vi "KH TURCK ETHERNETIP Global.vi"() -> ()   [LabVIEW 2017]
uses:
  KH TURCK ETHERNETIP TDefCluster TBEN-S2-4AI Input Values.ctl
  KH TURCK ETHERNETIP TDefCluster TBEN-S1-8DXP Input Values.ctl
  KH TURCK ETHERNETIP TDefCluster TBEN-S2-2RFID-4DXP Input Values.ctl
  KH TURCK ETHERNETIP TDefCluster TBEN-S2-4AO Input Values.ctl
  KH TURCK ETHERNETIP TDef Enum IOL Data.ctl
panel:
  in  "Tab Control 2":enum32{"AI", "DXP", "RFID", "AO", "IOL"}(tab)
  out "Read AI":T1[](array[typedef])
  out "Read DXP":T2[](array[typedef])
  out "RFID_Read":T3[](array[typedef])
  out "Data Turck":u8[](array[numeric]) format="%.0x"
  out "Read AO":T4[](array[typedef])
  out "Read IOL":T5[](array[typedef])
  # "Wire Break"
  # "upper limit"
  # "Overflow"
  # "Underflow"
  # "CJC Wire Break"
  # "Overcurrent (RTD)"
  # "Overcurrent supply VAUX1"
  # "Lower limit value underrun"
  # "Ch0"
  # "Ch1"
  # "Ch2"
  # "Ch3"
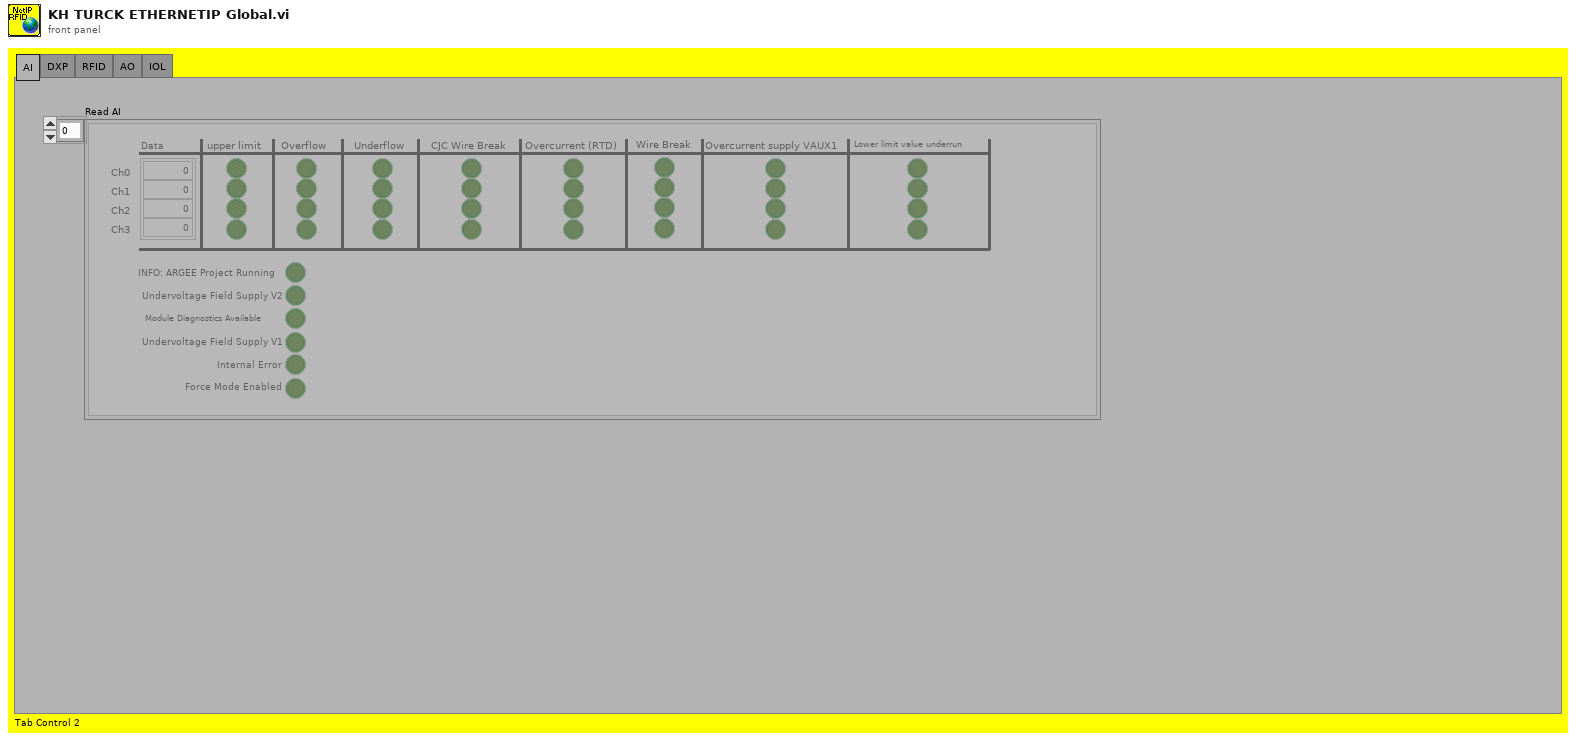
[diagram p1: front panel]
types:
  T1 = typedef "KH TURCK ETHERNETIP TDefCluster TBEN-S2-4AI Input Values.ctl" = cluster{"Data":i16[], "upper Limit CH0":bool, "upper Limit CH1":bool, "upper Limit CH2":bool, "upper Limit CH3":bool, "Overflow CH0":bool, "Overflow CH1":bool, "Overflow CH2":bool, "Overflow CH3":bool, "Underflow CH0":bool, "Underflow CH1":bool, "Underflow CH2":bool, "Underflow CH3":bool, "CJC Wire Break CH0":bool, "CJC Wire Break CH1":bool, "CJC Wire Break CH2":bool, "CJC Wire Break CH3":bool, "Overcurrent (RTD) CH0":bool, "Overcurrent (RTD) CH1":bool, "Overcurrent (RTD) CH2":bool, "Overcurrent (RTD) CH3":bool, "Wire Break CH0":bool, "Wire Break CH1":bool, "Wire Break CH2":bool, "Wire Break CH3":bool, "Overcurrent supply VAUX1 CH0":bool, "Overcurrent supply VAUX1 CH1":bool, "Overcurrent supply VAUX1 CH2":bool, "Overcurrent supply VAUX1 CH3":bool, "Lower limit value underrun CH0":bool, "Lower limit value underrun CH1":bool, "Lower limit value underrun CH2":bool, "Lower limit value underrun CH3":bool, "Module Diagnostics Available":bool, "INFO: ARGEE Project Running":bool, "Undervoltage Field Supply V2":bool, "Undervoltage Field Supply V1":bool, "Internal Error":bool, "Force Mode Enabled":bool}
  T2 = typedef "KH TURCK ETHERNETIP TDefCluster TBEN-S1-8DXP Input Values.ctl" = cluster{"Data":bool[], "Overcurrent":bool[], "Overcurrent VAUX1 Ch0-3":bool, "Overcurrent VAUX2 Ch4-7":bool, "Latch Input":bool[], "Counter value":u32, "Counter frequency (Hz)":u16, "Status":u8, "Overcurrent PWM Output 3":u8, "Overcurrent PWM Output 7":u8, "Module Diagnostics Available":bool, "INFO: ARGEE Project Running":bool, "Undervoltage V2":bool, "Undervoltage V1":bool, "Force Mode Enabled":bool}
  T3 = typedef "KH TURCK ETHERNETIP TDefCluster TBEN-S2-2RFID-4DXP Input Values.ctl" = cluster{"Station Status Word (Input Data Mapping)":cluster{"Module diagnostics avaliable":bool, "INFO: ARGEE Project Running":bool, "Undervoltage V2":bool, "Undervoltage V1":bool, "Internal Error":bool, "I/O-ASSISTANT Force Mode active":bool}, "RFID control/status 0 (Input Data Mapping)":cluster{"Tag present at r/w head":bool[], "response code":u16, "loop counter":u8, "Length":u16, "Error code":u16, "Tag counter":u16, "Data (Bytes) available":u16, "Read fragment No.":u8, "Write fragment No.":u8, "Tag present at r/w head bit":bool, "HF r/w head switched on":bool, "Continuous mode active":bool, "Antenna detuned at HF read/write head":bool, "Parameter not supported by read/write head":bool, "Error reported by read/write head":bool, "Not connected to read/write head":bool}, "RFID read data 0 (Input Data Mapping)":u8[], "RFID control/status 1 (Input Data Mapping)":cluster{"response code":u16, "Loop counter":u8, "Length":u16, "Error code":u16, "Tag counter":u16, "Data (Bytes) available":u16, "Read fragment No.":u8, "Write fragment No.":u8, "Tag present at r/w head bit":bool, "HF r/w head switched on":bool, "Continuous mode active":bool, "Antenna detuned at HF read/write head":bool, "Parameter not supported by read/write head":bool, "Error reported by read/write head":bool, "Not connected to read/write head":bool, "Tag present at r/w head":bool[]}, "RFID read data 1 (Input Data Mapping)":u8[], "RFID diagnostics (Input Data Mapping)":cluster{"Overcurrent supply VAUX1 (a)":bool, "Parameterization error (a)":bool, "Configuration via DTM active (a)":bool, "Buffer full (a)":bool, "Antenna detuned at HF read/write head (a)":bool[], "Parameter not supported by read/write head (a)":bool[], "Error reported by read/write head (a)":bool[], "Not connected to read/write head (a)":bool[], "Overcurrent supply VAUX1 (b)":bool, "Parameterization error (b)":bool, "Configuration via DTM active (b)":bool, "Buffer full (b)":bool, "Antenna detuned at HF read/write head (b)":bool[], "Parameter not supported by read/write head (b)":bool[], "Error reported by read/write head (b)":bool[], "Not connected to read/write head (b)":bool[]}, "DXP diagnostics (Input Data Mapping)":cluster{"Overcurrent VAUX2 Ch4/5":bool, "Overcurrent VAUX2 Ch6/7":bool, "Channel 4 - Output overcurrent":bool, "Channel 5 - Output overcurrent":bool, "Channel 6 - Output overcurrent":bool, "Channel 7 - Output overcurrent":bool}, "DXP (Input Data Mapping)":cluster{"Channel 4 - Input value":bool, "Channel 5 - Input value":bool, "Channel 6 - Input value":bool, "Channel 7 - Input value":bool}}
  T4 = typedef "KH TURCK ETHERNETIP TDefCluster TBEN-S2-4AO Input Values.ctl" = cluster{"Overload Ch0":bool, "Overload Ch1":bool, "Overload Ch2":bool, "Overload Ch3":bool, "Wirebreak Ch0":bool, "Wirebreak Ch1":bool, "Wirebreak Ch2":bool, "Wirebreak Ch3":bool, "Module Diagnostics Available":bool, "INFO: ARGEE Project Running":bool, "Undervoltage V2":bool, "Undervoltage V1":bool, "Internal Error":bool, "Force Mode Enabled":bool}
  T5 = typedef "KH TURCK ETHERNETIP TDef Enum IOL Data.ctl" = cluster{"Data_Port1":u16[], "Data_Port2":u16[], "Data_Port3":u16[], "Data_Port4":u16[], "Status":cluster{"Undervoltage Field Supply V2":bool, "Overvoltage Field Supply V1":bool, "Undervoltage Field Supply V1":bool, "Internal Error":bool, "Module Diagnostics Available":bool, "Station Configuration Changed":bool, "Overcurrent Isys":bool, "Overvoltage Field Supply V2":bool, "Force Mode Enabled":bool}, "Diagnostics":cluster{"Channel 2 - Output signal overcurrent":bool, "Channel 4 - Output signal overcurrent":bool, "Channel 6 - Output signal overcurrent":bool, "Channel 8 - Output signal overcurrent":bool, "Channel 1 - Wrong or missing device":bool, "Channel 3 - Wrong or missing device":bool, "Channel 5 - Wrong or missing device":bool, "Channel 7 - Wrong or missing device":bool, "Channel 1 - Data storage error":bool, "Channel 3 - Data storage error":bool, "Channel 5 - Data storage error":bool, "Channel 7 - Data storage error":bool, "Channel 1 - Process input data invalid":bool, "Channel 3 - Process input data invalid":bool, "Channel 5 - Process input data invalid":bool, "Channel 7 - Process input data invalid":bool, "Channel 1 - Hardware error":bool, "Channel 3 - Hardware error":bool, "Channel 5 - Hardware error":bool, "Channel 7 - Hardware error":bool, "Channel 1 - Maintenance events":bool, "Channel 3 - Maintenance events":bool, "Channel 5 - Maintenance events":bool, "Channel 7 - Maintenance events":bool, "Channel 1 - Out of spec. error":bool, "Channel 3 - Out of spec. error":bool, "Channel 5 - Out of spec. error":bool, "Channel 7 - Out of spec. error":bool, "Channel 1 - Parameterization error":bool, "Channel 3 - Parameterization error":bool, "Channel 5 - Parameterization error":bool, "Channel 1 - Overtemperature":bool, "Channel 3 - Overtemperature":bool, "Channel 5 - Overtemperature":bool, "Channel 7 - Overtemperature":bool, "Channel 1 - Lower limit value underrun":bool, "Channel 3 - Lower limit value underrun":bool, "Channel 5 - Lower limit value underrun":bool, "Channel 7 - Lower limit value underrun":bool, "Channel 1 - Upper limit value exceeded":bool, "Channel 3 - Upper limit value exceeded":bool, "Channel 5 - Upper limit value exceeded":bool, "Channel 7 - Upper limit value exceeded":bool, "Channel 1 - Undervoltage":bool, "Channel 3 - Undervoltage":bool, "Channel 5 - Undervoltage":bool, "Channel 7 - Undervoltage":bool, "Channel 1 - Overvoltage":bool, "Channel 3 - Overvoltage":bool, "Channel 5 - Overvoltage":bool, "Channel 7 - Overvoltage":bool, "Channel 1 - Overload":bool, "Channel 3 - Overload":bool, "Channel 5 - Overload":bool, "Channel 7 - Overload":bool, "Channel 1 - Common error":bool, "Channel 3 - Common error":bool, "Channel 5 - Common error":bool, "Channel 7 - Common error":bool, "Channel 1 - Port parameterization error":bool, "Channel 3 - Port parameterization error":bool, "Channel 5 - Port parameterization error":bool, "Channel 7 - Parameterization error":bool, "Channel 7 - Port parameterization error":bool}, "Events":cluster{"Event":u8[], "Qualifier":u8[], " Event code":u16[]}, "DXP":cluster{"DI Input value 2":bool, "DI Input value 4":bool, "DI Input value 6":bool, "DI Input value 8":bool, "DI Input 1":bool, "DI Input 3":bool, "DI Input 5":bool, "DI Input 7":bool, "Input values valid 1":bool, "Input values valid 3":bool, "Input values valid 5":bool, "Input values valid 7":bool}}
diagram:
